vi "templates LAYOUT data keys.vi"(6 "Template Record":T1, 9 "Template Keys":T2, 10 "HTM Keys":T2) -> (2 "HTM Keys":T2)   [LabVIEW 2011]
uses:
  Addons/internet/utils/keyedarr.llb/Keyed Array.ctl
  server/database/Templates/Template Record.ctl
  Addons/internet/utils/strutil.llb/Case Matching.ctl
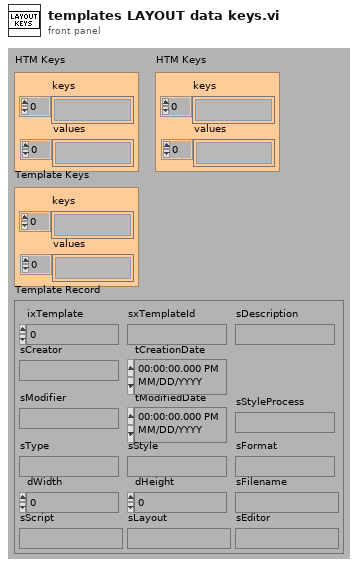
[diagram p1: front panel]
types:
  T1 = typedef "Template Record.ctl" = cluster{"ixTemplate":i32, "sxTemplateId":string, "sDescription":string, "sCreator":string, "tCreationDate":timestamp, "sModifier":string, "tModifiedDate":timestamp, "sType":string, "sStyle":string, "sFormat":string, "dWidth":dbl, "dHeight":dbl, "sFilename":string, "sScript":string, "sLayout":string, "sEditor":string, "sStyleProcess":string}
  T2 = typedef "Keyed Array.ctl" = cluster{"keys":string[], "values":string[]}
  T3 = typedef "Case Matching.ctl" = enum16{"a != A", "a == A", "system"}
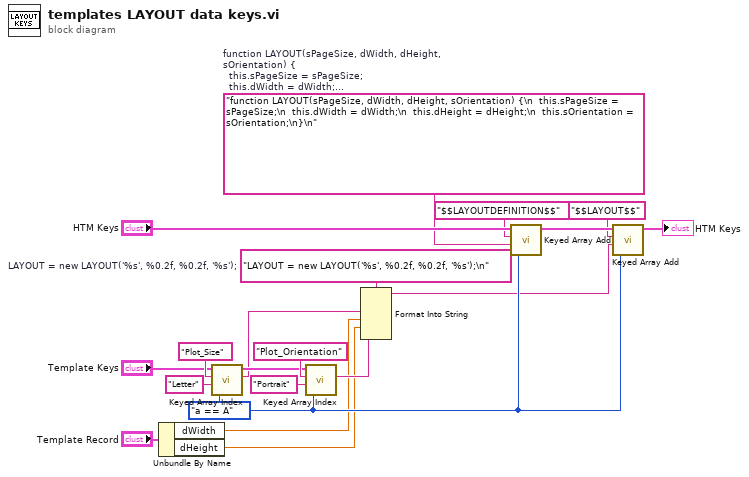
[diagram p0: block diagram]
diagram:
  w12 = "LAYOUT = new LAYOUT('%s', %0.2f, %0.2f, '%s');\n"  # LAYOUT = new LAYOUT('%s', %0.2f, %0.2f, '%s');
  w5 = Case_Matching."a == A" ("case matching (sensitive)")
  w18 = "function LAYOUT(sPageSize, dWidth, dHeight, sOrientation) {\n  this.sPageSize = sPageSize;\n  this.dWidth = dWidth;\n  this.dHeight = dHeight;\n  this.sOrientation = sOrientation;\n}\n"  # function LAYOUT(sPageSize, dWidth, dHeight, sOrientation) {   this.sPageSize = sPageSize;   this.dWidth = dWidth;   this.dHeight = dHeight;   this.sOrientation = sOrientation; }
  n1 = Unbundle By Name("Template Record") -> ("dWidth"=w2:dbl, "dHeight"=w1:dbl)
  n2 = call "Keyed Array Index.vi"("case matching (sensitive)"=w5, "default value"="Letter" ("key"), "key"="Plot_Size", "array in"="Template Keys") -> ("value"=w7:string, "duplicate array"=w9:T2)  [unwired: 2 out]
  n3 = call "Keyed Array Index.vi"("case matching (sensitive)"=w5, "default value"="Portrait" ("key"), "key"="Plot_Orientation", "array in"=w9) -> ("value"=w8:string)  [unwired: 3 out]
  n4 = Format Into String(format string=w12, w7, w2, w1, w8) -> (resulting string=w4:string)  [unwired: 2 in, 1 out]
  n5 = call "Keyed Array Add.vi"("case matching (sensitive)"=w5, "value"=w18, "key"="$$LAYOUTDEFINITION$$", "array in"="HTM Keys") -> ("array out"=w17:T2)  [unwired: 3 out]
  n6 = call "Keyed Array Add.vi"("case matching (sensitive)"=w5, "value"=w4, "key"="$$LAYOUT$$", "array in"=w17) -> ("array out"=→"HTM Keys":T2)  [unwired: 3 out]
